vi "CC Observation Queue GUI.vi"() -> ()   [LabVIEW 2024]
uses:
  Subsystems/SS cluster Script Status Queue.ctl
  typedefs/CC cluster Observation.ctl
  CC enum Observation Status.ctl
  Telescope/CC cluster Telescope Offsets.ctl
  typedefs/CC cluster Observation Dither Options.ctl
  typedefs/CC enum Dither Selection.ctl
  typedefs/CC cluster RA and DEC.ctl
  Subsystems/SS typedef cluster Instrument Command Queue Data.ctl
  CC cluster Script State.ctl
  CC cluster Observation Settings.ctl
  CC cluster Air Mass Data.ctl
  Logging/CC enum Current Values Action.ctl
  typedefs/CC cluster Script.ctl
  typedefs/CC Script Step.ctl
  typedefs/CC enum Script Action.ctl
  Scripts/CC Rd Wr Script Action.ctl
  typedefs/CC enum Alarm Action.ctl
  hk-channel-class/hk-channel-class/HK Table/HK Table.lvclass
panel:
  in  "Open Plots":bool
  in  "Air Mass Tool":bool
  out "Row":i32 caption="Next"
  in  "queue idle":string="TELESCOPE IDLE"
  in  "clean table":bool
  in  "Auto Step":bool
  in  "Stop":bool
  out "Queue Running":i16(slide) scale=-1.0..4.0
  in  "Pause Q":bool
  in  "Run Queue":bool
  in  "Close":bool
  out "Queue":i32(listbox)
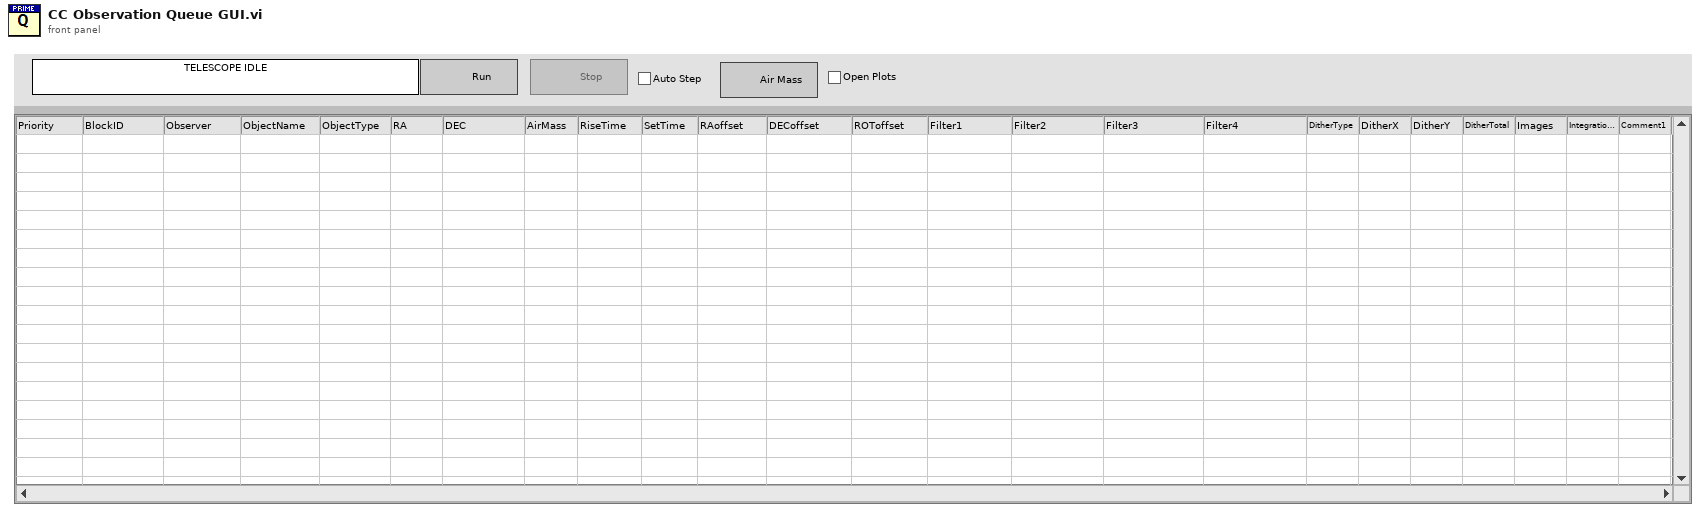
[diagram p1: front panel]
types:
  T1 = typedef "CC cluster Observation.ctl" = cluster{"Priority":i32, "ID":string, "Observer":string, "Obj Name":string, "Obj Type":string, "RA and DEC String":cluster{"RA":string, "DEC":string}, "Filters":string[], "Integration Time":dbl, "Observation Status":T2, "Offsets":T3, "Images":i32, "Dither Options":T4, "Comment 1":string, "Comment 2":string}
  T2 = typedef "CC enum Observation Status.ctl" = enum16{"Ready", "Running", "Done", "Error"}
  T3 = typedef "CC cluster Telescope Offsets.ctl" = cluster{"RA":dbl, "DEC":dbl, "ROT":dbl}
  T4 = typedef "CC cluster Observation Dither Options.ctl" = cluster{"Dither":T5, "Dither Radius":dbl, "Dither Points":i32, "Dither Phase":dbl, "B Offset":T6}
  T5 = typedef "CC enum Dither Selection.ctl" = enum16{"None", "Circle", "Random", "ABBA"}
  T6 = typedef "CC cluster RA and DEC.ctl" = cluster{"RA":dbl, "DEC":dbl}
  T7 = typedef "CC cluster Script State.ctl" = cluster{"Image Count":i32, "Step":i32, "Dither Idx":i32, "Dither Total":i32, "Running":bool, "State":u16}
  T8 = typedef "CC cluster Observation Settings.ctl" = cluster{"Air Mass Program Path":path}
  T9 = typedef "CC cluster Air Mass Data.ctl" = cluster{"BlockID":string, "Air Mass":string, "Rise Time":string, "Set Time":string}
  T10 = cluster{"state":refnum<user-event>, "Obs Queue":refnum<queue>, "Observation List":T1[], "Data":variant, "Obs State":enum16{"Idle", "Running", "Paused"}, "Row":i32, "Script Q":refnum<queue>, "Expected Images":i32, "Script Status":T7, "Prev Status":T7, "script name":string, "Observation Settings":T8, "BlockIDs":string[], "Airmass Idx":i32, "Air Mass":T9[]}
  T11 = typedef "CC enum Current Values Action.ctl" = enum16{"Init", "Write Item", "Write Array", "Read Item", "Read Array", "Read All", "Add Channels", "New File", "Add Message", "Get Current Values", "Close"}
  T12 = enum8{"Enabled", "Disabled", "Disabled and Grayed Out"}
  T13 = typedef "CC Rd Wr Script Action.ctl" = enum16{"Read", "Write", "List", "Delete"}
  T14 = typedef "CC cluster Script.ctl" = cluster{"Name":string, "Script":T15[]}
  T15 = typedef "CC Script Step.ctl" = cluster{"Action":T16, "Data":variant}
  T16 = typedef "CC enum Script Action.ctl" = enum16{"Noop", "Define Object", "Define Exposure", "Define Dithering", "Acquire Images", "Set Filter Wheel", "Telescope Home", "Telescope Move", "Telescope RA DEC", "Focus Move Relative", "Focus Move Absolute", "Focus Set Home", "Macro", "Pause", "Ask User", "Define Random Dither", "CmdLine", "Outlet"}
  T17 = typedef "SS typedef cluster Instrument Command Queue Data.ctl" = cluster{"Cmd":string, "Parameters":variant}
  T18 = typedef "CC enum Alarm Action.ctl" = enum16{"Init", "Add Alarm", "Get Alarms", "Clear Alarm", "Clear All Alarms"}
  T19 = typedef "SS cluster Script Status Queue.ctl" = cluster{"Msg":string, "Data":variant}
  T20 = typedef "CC cluster Script Panel Defaults.ctl" = cluster{"Script Name":string, "Script Path":path}
  T21 = typedef "LVPoint32TypeDef.ctl" = cluster{"Horizontal":i32, "Vertical":i32}
  T22 = typedef "LVRowAndColumnTypeDef.ctl" = cluster{"Row":i32, "Column":i32}
  T23 = typedef "CC cluster Alarm Data.ctl" = cluster{"Measured Value":dbl, "Alarm Low":dbl, "Alarm High":dbl, "Message":string, "Source":string}
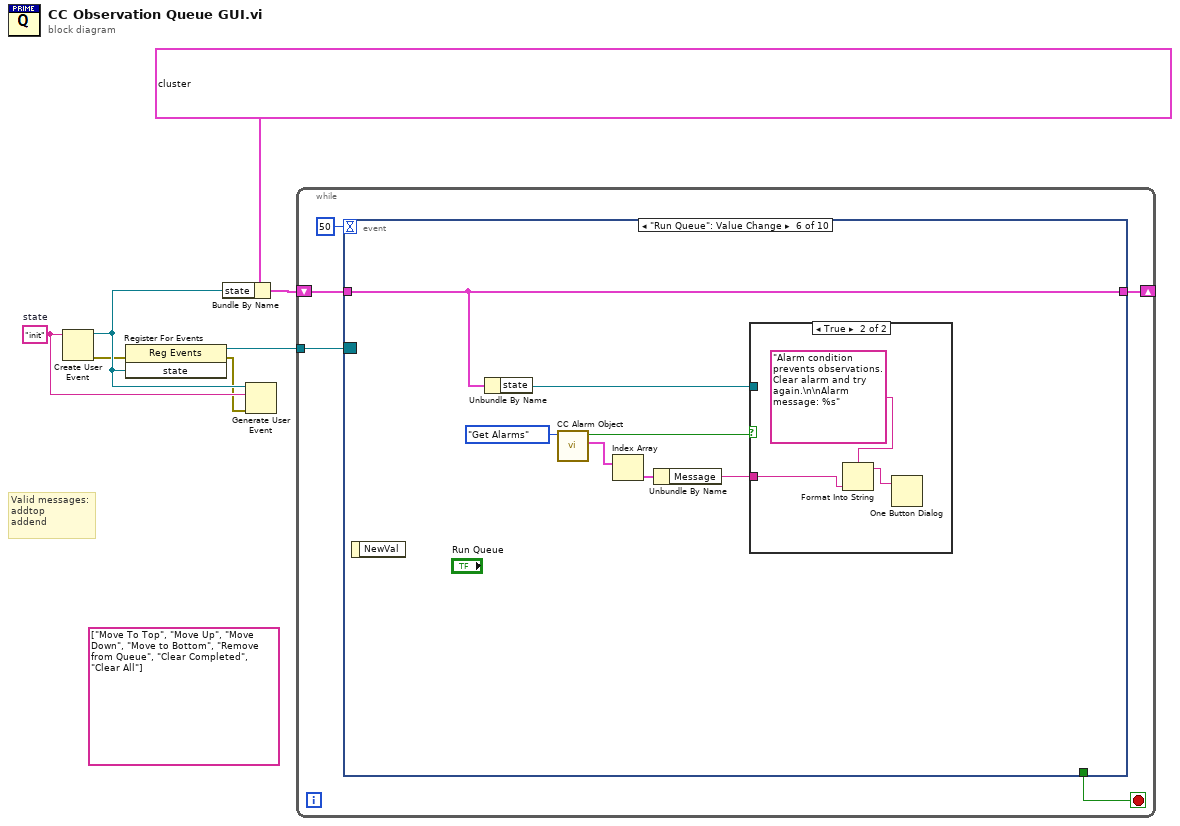
[diagram p0: block diagram]
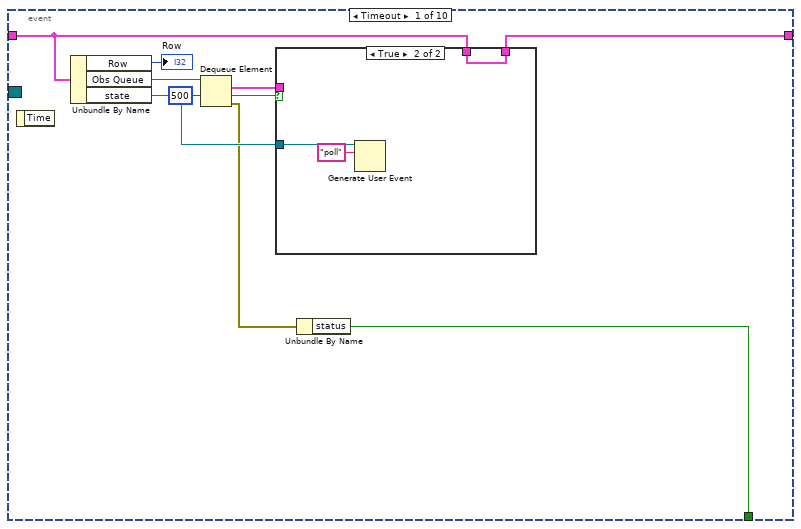
[diagram p2: hidden frame]
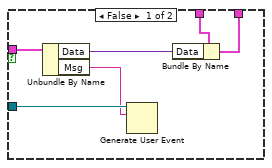
[diagram p3: hidden frame]
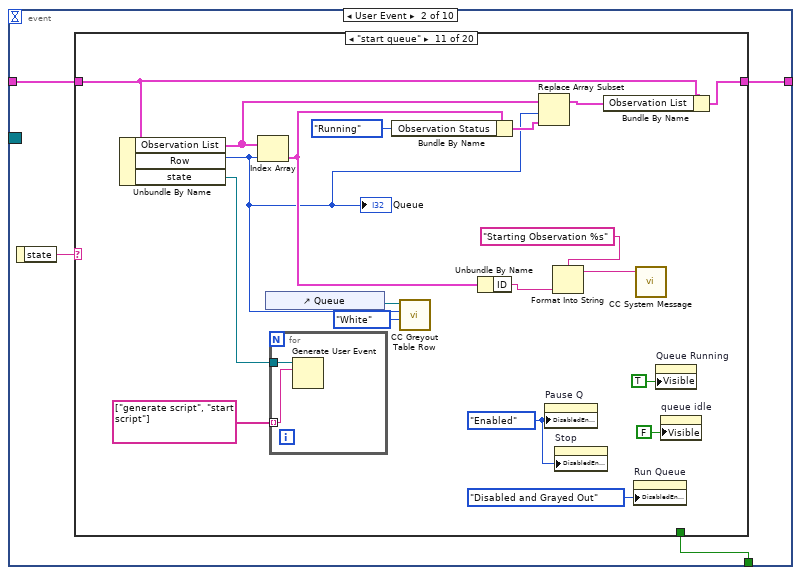
[diagram p4: hidden frame]
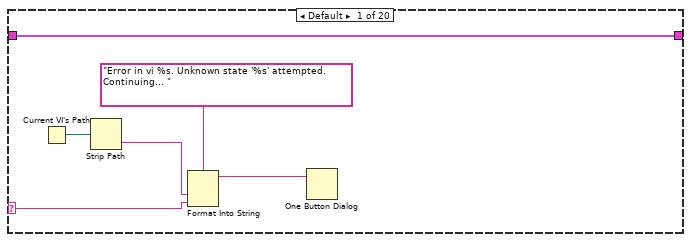
[diagram p5: hidden frame]
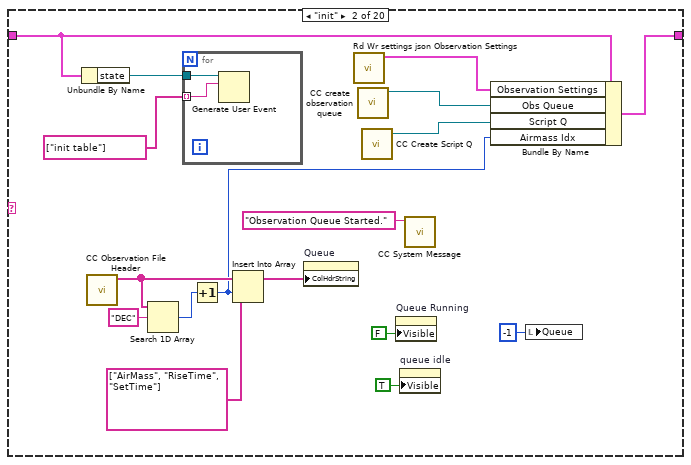
[diagram p6: hidden frame]
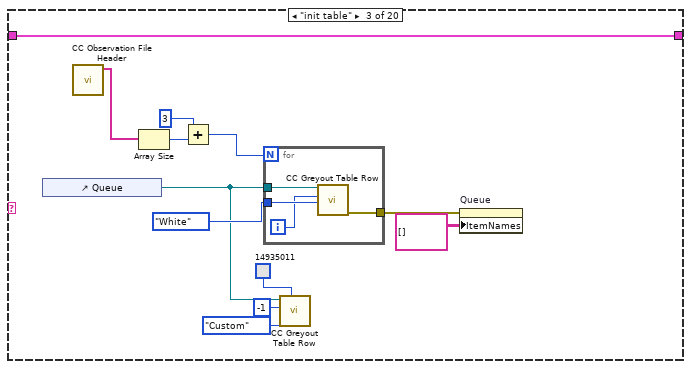
[diagram p7: hidden frame]
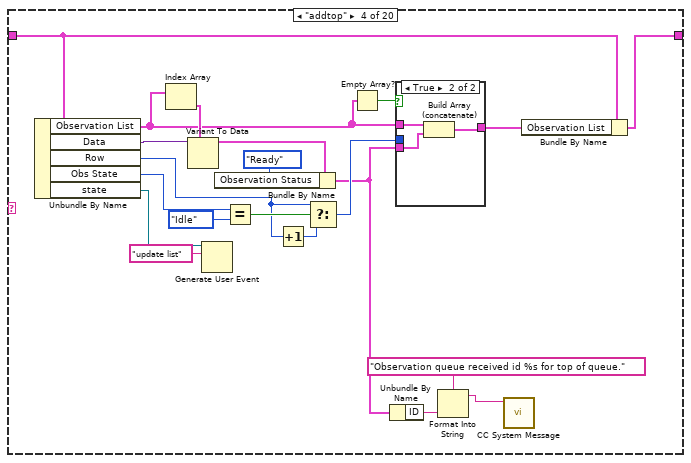
[diagram p8: hidden frame]
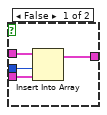
[diagram p9: hidden frame]
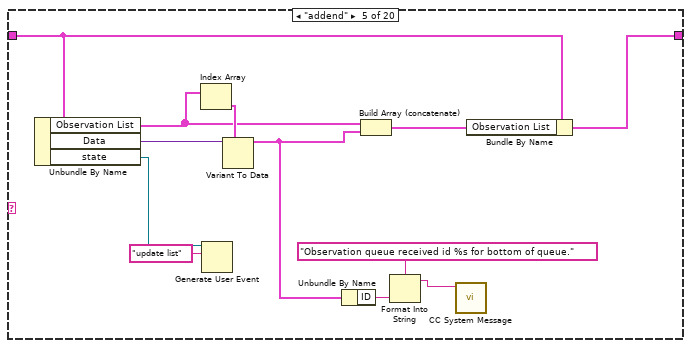
[diagram p10: hidden frame]
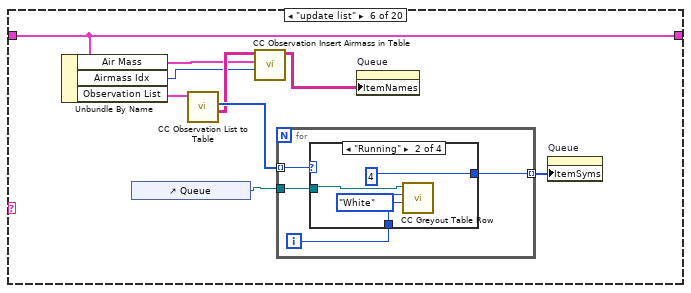
[diagram p11: hidden frame]
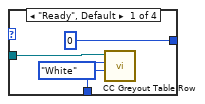
[diagram p12: hidden frame]
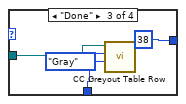
[diagram p13: hidden frame]
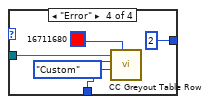
[diagram p14: hidden frame]
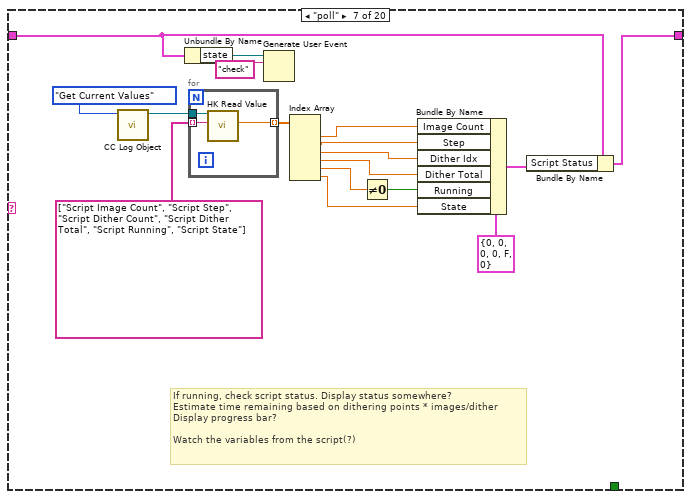
[diagram p15: hidden frame]
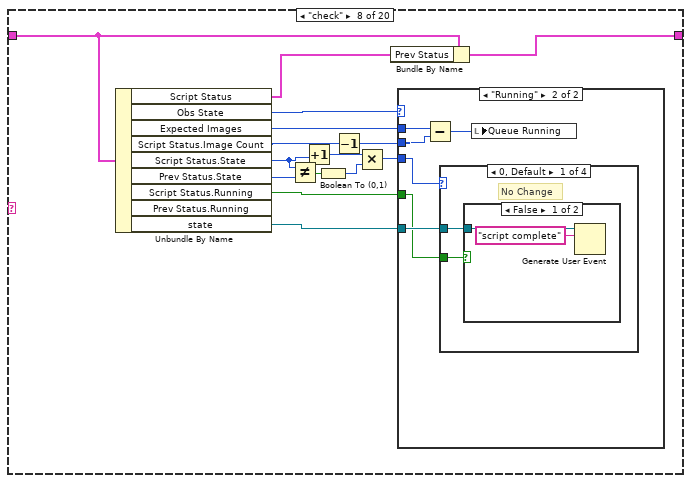
[diagram p16: hidden frame]
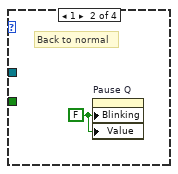
[diagram p19: hidden frame]
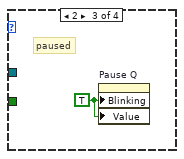
[diagram p20: hidden frame]
diagram:
  (unwired) string[] ["Move To Top", "Move Up", "Move Down", "Move to Bottom", "Remove from Queue", "Clear Completed", "Clear All"]
  w3 = "init"  # state
  # "Valid messages:\naddtop\naddend"
  n1 = Create User Event(user event datatype=w3) -> (user event=w5:refnum<user-event>, error out=w1:errorcluster)  [unwired: 1 in]
  n2 = register-events(error in=w1, w5) -> (reference out=w4:refnum<event-registration>, error out=w2:errorcluster)  [unwired: 1 in]
  n3 = Bundle By Name(cluster=T10 {"state"=refnum, "Obs Queue"=refnum, "Observation List"=[], "Data"=variant, "Obs State"=enum."Idle", "Row"=0, "Script Q"=refnum, "Expected Images"=0, "Script Status"={"Image Count"=0, "Step"=0, "Dither Idx"=0, "Dither Total"=0, "Running"=FALSE, "State"=0}, "Prev Status"={"Image Count"=0, "Step"=0, "Dither Idx"=0, "Dither Total"=0, "Running"=FALSE, "State"=0}, "script name"="", "Observation Settings"={"Air Mass Program Path"=path ""}, "BlockIDs"=["P0102", "P00002", "P00003", "P00004", "P00005", "P00006"], "Airmass Idx"=0, "Air Mass"=[{"BlockID"="", "Air Mass"="", "Rise Time"="06:16", "Set Time"="13:33"}, {"BlockID"="", "Air Mass"="", "Rise Time"="06:16", "Set Time"="13:33"}, {"BlockID"="", "Air Mass"="", "Rise Time"="06:16", "Set Time"="13:33"}, {"BlockID"="", "Air Mass"="", "Rise Time"="06:16", "Set Time"="13:33"}, {"BlockID"="", "Air Mass"="", "Rise Time"="06:16", "Set Time"="13:33"}, {"BlockID"="", "Air Mass"="", "Rise Time"="06:16", "Set Time"="13:33"}]}, "state"=w5) -> (w6:T10)
  n4 = Generate User Event(user event=w5, event data cluster=w3, error in=w2) -> ()  [unwired: 1 in, 2 out]
  n5 = while {
    tunnel: w4 -> [w12]
    shift-right: [w10] -> _
    shift-left: w6 -> [w11]
    stop <- w9 stop-if-true
    n6 = event shown="[5] \"Run Queue\": Value Change" {
      selector: w12 -> [_ _ _ _ _ _ _ _ _ _]
      dyn-events: _ -> [_ _ _ _ _ _ _ _ _ _]
      timeout: 50 -> [_ _ _ _ _ _ _ _ _ _]
      tunnel: w11 -> [w17 w34 w400 w432 w501 w578 w589 w594 w598 w600]
      tunnel: [w18 w33 w401 w432 w502 w578 w589 w594 w598 w600] -> w10
      tunnel: [w14 w32 _ _ _ _ _ _ _ "Close"] -> w9
      event Timeout {
        n7 = event-data() -> ()  [unwired: 1 in, 1 out]
        n8 = Unbundle By Name(w17) -> ("Row"=→"Row":i32, "Obs Queue"=w22:refnum<queue>, "state"=w19:refnum<user-event>)
        n9 = Dequeue Element(queue=w22, timeout in ms (-1)=500) -> (element=w20:T19, timed out?=w21:bool, error out=w15:errorcluster)  [unwired: 1 in, 1 out]
        n10 = case shown="True" w21 {
          tunnel: w20 -> [w28 _]
          tunnel: w19 -> [w27 w30]
          tunnel: w17 -> [w25 w31]
          tunnel: [w23 w31] -> w18
          frame False {
            n11 = Unbundle By Name(w28) -> ("Data"=w24:variant, "Msg"=w26:string)
            n12 = Generate User Event(user event=w27, event data cluster=w26) -> ()  [unwired: 2 in, 2 out]
            n13 = Bundle By Name(cluster=w25, "Data"=w24) -> (w23:T10)
          }
          frame True {
            n14 = Generate User Event(user event=w30, event data cluster="poll" ("event data")) -> ()  [unwired: 2 in, 2 out]
          }
        }
        n15 = Unbundle By Name(w15) -> ("status"=w14:bool)
      }
      event User Event {
        n16 = event-data() -> ("state"=w35:string)  [unwired: 1 in]
        n17 = case shown="\"start queue\"" w35 {
          selector: w35 -> [w40 _ _ _ _ _ _ _ _ _ _ _ _ _ _ _ _ _ _ _]
          tunnel: w34 -> [w36 w54 w72 w93 w111 w125 w150 w168 w202 w228 w232 w255 w293 w316 w337 w357 w366 w382 w392 w397]
          tunnel: [w36 w57 w72 w94 w112 w125 w151 w169 w203 w229 w233 w256 w304 w317 w338 w357 w367 w383 w392 w397] -> w33
          tunnel: [_ _ _ _ _ _ _ _ _ _ _ _ _ _ _ _ _ _ _ TRUE] -> w32
          frame Default {
            n18 = Current VI's Path() -> (path=w39:path)
            n19 = Strip Path(path=w39) -> (name=w38:string)  [unwired: 1 out]
            n20 = Format Into String(format string="Error in vi %s. Unknown state '%s' attempted. Continuing... ", w38, w40) -> (resulting string=w37:string)  [unwired: 2 in, 1 out]
            n21 = One Button Dialog(message=w37) -> ()  [unwired: 1 in, 1 out]
          }
          frame "init" {
            n22 = Unbundle By Name(w54) -> ("state"=w53:refnum<user-event>)
            n23 = call "CC Observation File Header.vi"() -> ("Header"=w47:string[])  [unwired: 10 in, 1 out]
            n24 = Search 1D Array(1D array=w47, element="DEC") -> (index of element=w44:i32)  [unwired: 1 in]
            n25 = for {
              tunnel: w53 -> [w60]
              tunnel: string[] ["init table"] -> [w59] mode=indexing
              n26 = Generate User Event(user event=w60, event data cluster=w59) -> ()  [unwired: 2 in, 2 out]
            }
            n27 = Increment(x=w44) -> (x+1=w42:i32)
            n28 = Insert Into Array(array=w47, index=w42, new element=string[] ["AirMass", "RiseTime", "SetTime"]) -> (w45:string[])
            n29 = property on="Queue" class="MCListbox (strict)"("ColHdrString"=w45) -> ()  [unwired: 2 in, 2 out]
            n30 = call "Rd Wr settings json Observation Settings.vi"() -> ("Observation Settings"=w48:T8)  [unwired: 10 in, 1 out]
            n31 = call "CC create observation queue.vi"() -> ("Observation Queue"=w58:refnum<queue>)  [unwired: 10 in, 1 out]
            n32 = call "CC Create Script Q.vi"() -> ("Script Q"=w56:refnum<queue>)  [unwired: 10 in, 1 out]
            n33 = property on="Queue Running" class="Slide (strict)"("Visible"=FALSE) -> ()  [unwired: 2 in, 2 out]
            n34 = property on="queue idle" class="Str"("Visible"=TRUE) -> ()  [unwired: 2 in, 2 out]
            n35 = call "CC System Message.vi"("Message"="Observation Queue Started.") -> ()  [unwired: 10 in, 1 out]
            n36 = Bundle By Name(cluster=w54, "Observation Settings"=w48, "Obs Queue"=w58, "Script Q"=w56, "Airmass Idx"=w42) -> (w57:T10)
            n37 = local write "Queue"(-1 ("Queue")) -> ()
          }
          frame "init table" {
            n38 = control-ref of="Queue"() -> (w68:refnum<vi>)
            n39 = call "CC Observation File Header.vi"() -> ("Header"=w64:string[])  [unwired: 10 in, 1 out]
            n40 = Array Size(array=w64) -> (size(s)=w63:i32)
            n41 = Add(x=3, y=w63) -> (x+y=w62:i32)
            n42 = for {
              N: w62 -> [_]
              tunnel: w68 -> [w76]
              tunnel: [w75] -> w71
              tunnel: enum16{"White", "Gray", "Custom"}."White" ("Color") -> [w74]
              i -> [w73]
              n43 = call "CC Greyout Table Row.vi"("Color"=w74, "Row"=w73, "Queue ref"=w76) -> ("error out"=w75:errorcluster)  [unwired: 8 in]
            }
            n44 = call "CC Greyout Table Row.vi"("Color Box"=u32 14935011, "Color"=enum16{"White", "Gray", "Custom"}."Custom", "Row"=-1, "Queue ref"=w68) -> ()  [unwired: 7 in, 1 out]
            n45 = property on="Queue" class="MCListbox (strict)"(error in=w71, "ItemNames"=string[][] [] ("Item Names")) -> ()  [unwired: 1 in, 2 out]
          }
          frame "addtop" {
            n46 = Unbundle By Name(w93) -> ("Observation List"=w82:T1[], "Data"=w97:variant, "Row"=w77:i32, "Obs State"=w92:enum16{"Idle", "Running", "Paused"}, "state"=w87:refnum<user-event>)
            n47 = Index Array(array=w82) -> (element=w96:T1)  [unwired: 1 in]
            n48 = Variant To Data(type=w96, Variant=w97) -> (data=w81:T1)  [unwired: 1 in, 1 out]
            n49 = Generate User Event(user event=w87, event data cluster="update list" ("event data")) -> ()  [unwired: 2 in, 2 out]
            n50 = Bundle By Name(cluster=w81, "Observation Status"=CC_enum_Observation_Status."Ready") -> (w79:T1)
            n51 = Equal?(x=w92, y=enum16{"Idle", "Running", "Paused"}."Idle") -> (x = y?=w90:bool)
            n52 = Increment(x=w77) -> (x+1=w88:i32)
            n53 = Select(t=w77, s=w90, f=w88) -> (s? t:f=w89:i32)
            n54 = Empty Array?(array=w82) -> (empty?=w78:bool)
            n55 = Unbundle By Name(w79) -> ("ID"=w84:string)
            n56 = case shown="True" w78 {
              tunnel: [w101 w102] -> w95
              tunnel: w89 -> [w100 _]
              tunnel: w82 -> [w99 w104]
              tunnel: w79 -> [w98 w103]
              frame False {
                n57 = Insert Into Array(array=w99, index=w100, new element=w98) -> (w101:T1[])
              }
              frame True {
                n58 = Build Array (concatenate)(w104, w103) -> (w102:T1[])
              }
            }
            n59 = Format Into String(format string="Observation queue received id %s for top of queue.", w84) -> (resulting string=w83:string)  [unwired: 2 in, 1 out]
            n60 = call "CC System Message.vi"("Message"=w83) -> ()  [unwired: 10 in, 1 out]
            n61 = Bundle By Name(cluster=w93, "Observation List"=w95) -> (w94:T10)
          }
          frame "addend" {
            n62 = Unbundle By Name(w111) -> ("Observation List"=w114:T1[], "Data"=w116:variant, "state"=w110:refnum<user-event>)
            n63 = Index Array(array=w114) -> (element=w115:T1)  [unwired: 1 in]
            n64 = Generate User Event(user event=w110, event data cluster="update list" ("event data")) -> ()  [unwired: 2 in, 2 out]
            n65 = Variant To Data(type=w115, Variant=w116) -> (data=w105:T1)  [unwired: 1 in, 1 out]
            n66 = Unbundle By Name(w105) -> ("ID"=w107:string)
            n67 = Build Array (concatenate)(w114, w105) -> (w113:T1[])
            n68 = Format Into String(format string="Observation queue received id %s for bottom of queue.", w107) -> (resulting string=w106:string)  [unwired: 2 in, 1 out]
            n69 = call "CC System Message.vi"("Message"=w106) -> ()  [unwired: 10 in, 1 out]
            n70 = Bundle By Name(cluster=w111, "Observation List"=w113) -> (w112:T10)
          }
          frame "update list" {
            n71 = Unbundle By Name(w125) -> ("Air Mass"=w119:T9[], "Airmass Idx"=w118:i32, "Observation List"=w124:T1[])
            n72 = control-ref of="Queue"() -> (w121:refnum<vi>)
            n73 = call "CC Observation List to Table.vi"("Observation List"=w124) -> ("Screen Ready Table"=w120:string[][], "Status"=w123:T2[])  [unwired: 7 in, 2 out]
            n74 = call "CC Observation Insert Airmass in Table.vi"("Airmass Idx"=w118, "Air Mass"=w119, "Table"=w120) -> ("Table out"=w117:string[][])  [unwired: 8 in]
            n75 = for {
              tunnel: w123 -> [w129] mode=indexing
              tunnel: [w128] -> w122 mode=indexing
              tunnel: w121 -> [w126]
              i -> [w127]
              n76 = case shown="\"Running\"" w129 {
                tunnel: [0 4 ("new element/subarray") 38 ("new element/subarray") 2 ("new element/subarray")] -> w128
                tunnel: w127 -> [w132 w137 w140 w143]
                tunnel: w126 -> [w130 w136 w139 w145]
                frame "Ready", Default {
                  n77 = call "CC Greyout Table Row.vi"("Color"=enum16{"White", "Gray", "Custom"}."White", "Row"=w132, "Queue ref"=w130) -> ()  [unwired: 8 in, 1 out]
                }
                frame "Running" {
                  n78 = call "CC Greyout Table Row.vi"("Color"=enum16{"White", "Gray", "Custom"}."White", "Row"=w137, "Queue ref"=w136) -> ()  [unwired: 8 in, 1 out]
                }
                frame "Done" {
                  n79 = call "CC Greyout Table Row.vi"("Color"=enum16{"White", "Gray", "Custom"}."Gray", "Row"=w140, "Queue ref"=w139) -> ()  [unwired: 8 in, 1 out]
                }
                frame "Error" {
                  n80 = call "CC Greyout Table Row.vi"("Color Box"=u32 16711680, "Color"=enum16{"White", "Gray", "Custom"}."Custom", "Row"=w143, "Queue ref"=w145) -> ()  [unwired: 7 in, 1 out]
                }
              }
            }
            n81 = property on="Queue" class="MCListbox (strict)"("ItemNames"=w117) -> ()  [unwired: 2 in, 2 out]
            n82 = property on="Queue" class="MCListbox (strict)"("ItemSyms"=w122) -> ()  [unwired: 2 in, 2 out]
          }
          frame "poll" {
            # "If running, check script status. Display status somewhere?\nEstimate time remaining based on dithering points * images/dither\nDisplay progress bar?\n\nWatch the variables from the script(?)"
            n83 = call "CC Log Object.vi"("Action"=CC_enum_Current_Values_Action."Get Current Values") -> ("HK Channel out"=w162:refnum<class "HK Table.lvclass">)  [unwired: 8 in, 2 out]
            n84 = Unbundle By Name(w150) -> ("state"=w148:refnum<user-event>)
            n85 = for {
              tunnel: w162 -> [w166]
              tunnel: string[] ["Script Image Count", "Script Step", "Script Dither Count", "Script Dither Total", "Script Running", "Script State"] -> [w165] mode=indexing
              tunnel: [w164] -> w161 mode=indexing
              n86 = call-dynamic "HK Read Value.vi"("Channel Name"=w165, "HK Channel in"=w166) -> ("Value"=w164:dbl)  [unwired: 4 in, 5 out]
            }
            n87 = Generate User Event(user event=w148, event data cluster="check" ("event data")) -> ()  [unwired: 2 in, 2 out]
            n88 = Index Array(array=w161) -> (element #1=w149:dbl, element #2=w158:dbl, element #3=w157:dbl, element #4=w156:dbl, element #5=w155:dbl, element #6=w153:dbl)  [unwired: 6 in]
            n89 = Not Equal To 0?(x=w155) -> (x != 0?=w154:bool)
            n90 = Bundle By Name(cluster=T7 {"Image Count"=0, "Step"=0, "Dither Idx"=0, "Dither Total"=0, "Running"=FALSE, "State"=0}, "Image Count"=w149, "Step"=w158, "Dither Idx"=w157, "Dither Total"=w156, "Running"=w154, "State"=w153) -> (w152:T7)
            n91 = Bundle By Name(cluster=w150, "Script Status"=w152) -> (w151:T10)
          }
          frame "check" {
            n92 = Unbundle By Name(w168) -> ("Script Status"=w170:T7, "Obs State"=w181:enum16{"Idle", "Running", "Paused"}, "Expected Images"=w180:i32, "Script Status.Image Count"=w179:i32, "Script Status.State"=w177:u16, "Prev Status.State"=w178:u16, "Script Status.Running"=w171:bool, "state"=w172:refnum<user-event>)  [unwired: 1 out]
            n93 = Not Equal?(x=w177, y=w178) -> (x != y?=w175:bool)
            n94 = Increment(x=w177) -> (x+1=w176:u16)
            n95 = Boolean To (0,1)(Boolean=w175) -> (0, 1=w173:i16)
            n96 = Decrement(x=w179) -> (x-1=w167:i32)
            n97 = Multiply(x=w176, y=w173) -> (x*y=w174:u16)
            n98 = Bundle By Name(cluster=w168, "Prev Status"=w170) -> (w169:T10)
            n99 = case shown="\"Running\"" w181 {
              tunnel: w180 -> [_ w187]
              tunnel: w167 -> [_ w185]
              tunnel: w174 -> [_ w184]
              tunnel: w172 -> [_ w183]
              tunnel: w171 -> [_ w182]
              frame "Idle", Default {
              }
              frame "Running" {
                n100 = Subtract(x=w187, y=w185) -> (x-y=w186:i32)
                n101 = case shown="0, Default" w184 {
                  tunnel: w183 -> [w189 _ _ w195]
                  tunnel: w182 -> [w188 _ _ _]
                  frame 0, Default {
                    # "No Change"
                    n102 = case shown="False" w188 {
                      tunnel: w189 -> [w190 _]
                      frame False {
                        n103 = Generate User Event(user event=w190, event data cluster="script complete" ("event data")) -> ()  [unwired: 2 in, 2 out]
                      }
                      frame True {
                      }
                    }
                  }
                  frame 1 {
                    w192 = FALSE ("Blinking")
                    # "Back to normal"
                    n104 = property on="Pause Q" class="Bool (strict)"("Blinking"=w192, "Value"=w192) -> ()  [unwired: 2 in, 2 out]
                  }
                  frame 2 {
                    w193 = TRUE ("Blinking")
                    # "paused"
                    n105 = property on="Pause Q" class="Bool (strict)"("Blinking"=w193, "Value"=w193) -> ()  [unwired: 2 in, 2 out]
                  }
                  frame 3 {
                    # "Error"
                    n106 = Generate User Event(user event=w195, event data cluster="script error" ("event data")) -> ()  [unwired: 2 in, 2 out]
                  }
                }
                n107 = local write "Queue Running"(w186) -> ()
              }
            }
          }
          frame "add to top" {
            n108 = Unbundle By Name(w202) -> ("Data"=w209:variant, "Obs State"=w208:enum16{"Idle", "Running", "Paused"}, "Row"=w207:i32, "Observation List"=w206:T1[], "state"=w201:refnum<user-event>)
            n109 = Variant To Data(type=T1 {"Priority"=0, "ID"="", "Observer"="", "Obj Name"="", "Obj Type"="", "RA and DEC String"={"RA"="", "DEC"=""}, "Filters"=[], "Integration Time"=0.0, "Observation Status"=enum."Error", "Offsets"={"RA"=0.0, "DEC"=0.0, "ROT"=0.0}, "Images"=0, "Dither Options"={"Dither"=enum."Random", "Dither Radius"=0.0, "Dither Points"=0, "Dither Phase"=0.0, "B Offset"={"RA"=0.0, "DEC"=0.0}}, "Comment 1"="", "Comment 2"=""} ("Observation"), Variant=w209) -> (data=w205:T1)  [unwired: 1 in, 1 out]
            n110 = Generate User Event(user event=w201, event data cluster="update list" ("event data")) -> ()  [unwired: 2 in, 2 out]
            n111 = case shown="\"Idle\", Default" w208 {
              tunnel: w207 -> [_ w219]
              tunnel: w206 -> [w214 w218]
              tunnel: w205 -> [w211 w215]
              tunnel: [w212 w216] -> w204
              tunnel: [w211 w215] -> w198
              frame "Idle", Default {
                n112 = Insert Into Array(array=w214, index=0, new element=w211) -> (w212:T1[])
              }
              frame "Running", "Paused" {
                n113 = Increment(x=w219) -> (x+1=w217:i32)
                n114 = Insert Into Array(array=w218, index=w217, new element=w215) -> (w216:T1[])
              }
            }
            n115 = Unbundle By Name(w198) -> ("ID"=w197:string)
            n116 = Format Into String(format string="Observation ID %s added to top of Queue" ("Message"), w197) -> (resulting string=w196:string)  [unwired: 2 in, 1 out]
            n117 = Bundle By Name(cluster=w202, "Observation List"=w204) -> (w203:T10)
            n118 = call "CC System Message.vi"("Message"=w196) -> ()  [unwired: 10 in, 1 out]
          }
          frame "add to bottom" {
            n119 = Unbundle By Name(w228) -> ("Data"=w230:variant, "Observation List"=w225:T1[], "state"=w227:refnum<user-event>)
            n120 = Variant To Data(type=T1 {"Priority"=0, "ID"="", "Observer"="", "Obj Name"="", "Obj Type"="", "RA and DEC String"={"RA"="", "DEC"=""}, "Filters"=[], "Integration Time"=0.0, "Observation Status"=enum."Error", "Offsets"={"RA"=0.0, "DEC"=0.0, "ROT"=0.0}, "Images"=0, "Dither Options"={"Dither"=enum."Random", "Dither Radius"=0.0, "Dither Points"=0, "Dither Phase"=0.0, "B Offset"={"RA"=0.0, "DEC"=0.0}}, "Comment 1"="", "Comment 2"=""} ("Observation"), Variant=w230) -> (data=w220:T1)  [unwired: 1 in, 1 out]
            n121 = Generate User Event(user event=w227, event data cluster="update list" ("event data")) -> ()  [unwired: 2 in, 2 out]
            n122 = Build Array (concatenate)(w225, w220) -> (w224:T1[])
            n123 = Unbundle By Name(w220) -> ("ID"=w222:string)
            n124 = Format Into String(format string="Observation ID %s added to end of Queue" ("Message"), w222) -> (resulting string=w221:string)  [unwired: 2 in, 1 out]
            n125 = Bundle By Name(cluster=w228, "Observation List"=w224) -> (w229:T10)
            n126 = call "CC System Message.vi"("Message"=w221) -> ()  [unwired: 10 in, 1 out]
          }
          frame "start queue" {
            w247 = T12."Enabled" ("Disabled")
            n127 = Unbundle By Name(w232) -> ("Observation List"=w237:T1[], "Row"=w235:i32, "state"=w249:refnum<user-event>)
            "Queue" <- w235
            n128 = Index Array(array=w237, index=w235) -> (element=w239:T1)
            n129 = control-ref of="Queue"() -> (w243:refnum<vi>)
            n130 = for {
              tunnel: w249 -> [w252]
              tunnel: string[] ["generate script", "start script"] -> [w251] mode=indexing
              n131 = Generate User Event(user event=w252, event data cluster=w251) -> ()  [unwired: 2 in, 2 out]
            }
            n132 = Bundle By Name(cluster=w239, "Observation Status"=CC_enum_Observation_Status."Running") -> (w236:T1)
            n133 = call "CC Greyout Table Row.vi"("Color"=enum16{"White", "Gray", "Custom"}."White", "Row"=w235, "Queue ref"=w243) -> ()  [unwired: 8 in, 1 out]
            n134 = Unbundle By Name(w239) -> ("ID"=w245:string)
            n135 = Replace Array Subset(array=w237, new element=w236, index=w235) -> (w234:T1[])
            n136 = property on="Pause Q" class="Bool (strict)"("DisabledEnum"=w247) -> ()  [unwired: 2 in, 2 out]
            n137 = Format Into String(format string="Starting Observation %s" ("Message"), w245) -> (resulting string=w244:string)  [unwired: 2 in, 1 out]
            n138 = property on="Stop" class="Bool"("DisabledEnum"=w247) -> ()  [unwired: 2 in, 2 out]
            n139 = Bundle By Name(cluster=w232, "Observation List"=w234) -> (w233:T10)
            n140 = property on="Run Queue" class="Bool"("DisabledEnum"=T12."Disabled and Grayed Out" ("Disabled")) -> ()  [unwired: 2 in, 2 out]
            n141 = call "CC System Message.vi"("Message"=w244) -> ()  [unwired: 10 in, 1 out]
            n142 = property on="Queue Running" class="Slide (strict)"("Visible"=TRUE) -> ()  [unwired: 2 in, 2 out]
            n143 = property on="queue idle" class="Str"("Visible"=FALSE) -> ()  [unwired: 2 in, 2 out]
          }
          frame "quick image" {
            n144 = Unbundle By Name(w255) -> ("state"=w253:refnum<user-event>, "Obs State"=w254:enum16{"Idle", "Running", "Paused"}, "Script Q"=w257:refnum<queue>, "Data"=w258:variant)
            n145 = case shown="\"Idle\"" w254 {
              tunnel: w258 -> [w281 _]
              tunnel: w257 -> [w277 _]
              tunnel: [w262 w283] -> w256
              tunnel: w255 -> [w261 w283]
              tunnel: w253 -> [w260 _]
              frame "Idle" {
                n146 = Variant To Data(type=T1 {"Priority"=0, "ID"="", "Observer"="", "Obj Name"="", "Obj Type"="", "RA and DEC String"={"RA"="HH:MM:SS.nnn", "DEC"="DEG:arcmin:arcsec.nn"}, "Filters"=[], "Integration Time"=0.0, "Observation Status"=enum."Error", "Offsets"={"RA"=0.0, "DEC"=0.0, "ROT"=0.0}, "Images"=0, "Dither Options"={"Dither"=enum."None", "Dither Radius"=0.0, "Dither Points"=0, "Dither Phase"=0.0, "B Offset"={"RA"=0.0, "DEC"=0.0}}, "Comment 1"="", "Comment 2"=""} ("element"), Variant=w281) -> (data=w275:T1)  [unwired: 1 in, 1 out]
                n147 = Format Date/Time String(time format string (%c)="%Y%m%d_%H%M%S") -> (date/time string=w265:string)  [unwired: 2 in]
                n148 = call "CC Observation to Script.vi"("Observation"=w275) -> ("Script Steps"=w264:T15[])  [unwired: 9 in, 1 out]
                n149 = call "Rd Wr Script Defaults.vi"() -> ("Script Settings"=w272:T20)  [unwired: 10 in, 1 out]
                n150 = Format Into String(format string="QuickObs_%s", w265) -> (resulting string=w263:string)  [unwired: 2 in, 1 out]
                n151 = Bundle(cluster=T17 {"Cmd"="", "Parameters"=variant} ("element"), "Cmd"="set observation", "Parameters"=w275) -> (w276:T17)
                n152 = Unbundle By Name(w272) -> ("Script Path"=w271:path)
                n153 = Bundle By Name(cluster=T14 {"Name"="", "Script"=[]} ("Script"), "Name"=w263, "Script"=w264) -> (w273:T14)
                n154 = Generate User Event(user event=w260, event data cluster="start script" ("event data")) -> ()  [unwired: 2 in, 2 out]
                n155 = Enqueue Element(queue=w277, element=w276) -> ()  [unwired: 2 in, 3 out]
                n156 = Bundle By Name(cluster=w261, "script name"=w263) -> (w262:T10)
                n157 = Format Into String(format string="Created script %s.", w263) -> (resulting string=w267:string)  [unwired: 2 in, 1 out]
                n158 = call "CC Rd Wr Script.vi"("Script Path"=w271, "Action"=CC_Rd_Wr_Script_Action."Write", "Script"=w273) -> ()  [unwired: 3 in, 6 out]
                n159 = call "CC System Message.vi"("Message"=w267) -> ()  [unwired: 10 in, 1 out]
              }
              frame "Running", Default {
                n160 = One Button Dialog(message="Cannot take a quick image right now. Image acquisition already underway.") -> ()  [unwired: 1 in, 1 out]
              }
            }
          }
          frame "generate script" {
            # "Name the script file from ID and Obj name"
            # "create the script file and send to script process but don't run it"
            n161 = Unbundle By Name(w293) -> ("Observation List"=w303:T1[], "Row"=w302:i32)
            n162 = property on="Queue" class="MCListbox (strict)"() -> ("ItemSyms"=w307:i32[])  [unwired: 2 in, 2 out]
            n163 = Unbundle By Name(w293) -> ("Script Q"=w285:refnum<queue>)
            n164 = local write "Queue"(w302) -> ()
            n165 = Replace Array Subset(array=w307, new element=4 ("new element/subarray"), index=w302) -> (w305:i32[])
            n166 = Index Array(array=w303, index=w302) -> (element=w286:T1)
            n167 = property on="Queue" class="MCListbox (strict)"("ItemSyms"=w305) -> ()  [unwired: 2 in, 2 out]
            n168 = call "CC Observation to Script.vi"("Observation"=w286) -> ("Script Steps"=w294:T15[])  [unwired: 9 in, 1 out]
            n169 = call "CC Observation Count Images.vi"("element"=w286) -> ("Total Images"=w290:i32)  [unwired: 9 in, 1 out]
            "Queue Running" <- w290
            n170 = Unbundle By Name(w286) -> ("ID"=w300:string)
            n171 = Bundle(cluster=T17 {"Cmd"="", "Parameters"=variant} ("element"), "Cmd"="set observation", "Parameters"=w286) -> (w287:T17)
            n172 = call "Rd Wr Script Defaults.vi"() -> ("Script Settings"=w298:T20)  [unwired: 10 in, 1 out]
            n173 = Format Into String(format string="Obs_%s", w300) -> (resulting string=w284:string)  [unwired: 2 in, 1 out]
            n174 = Enqueue Element(queue=w285, element=w287) -> ()  [unwired: 2 in, 3 out]
            n175 = Unbundle By Name(w298) -> ("Script Path"=w297:path)
            n176 = Bundle By Name(cluster=T14 {"Name"="", "Script"=[]} ("Script"), "Name"=w284, "Script"=w294) -> (w299:T14)
            n177 = Bundle By Name(cluster=w293, "Expected Images"=w290, "script name"=w284) -> (w304:T10)
            n178 = Format Into String(format string="Created script %s.", w284) -> (resulting string=w291:string)  [unwired: 2 in, 1 out]
            n179 = call "CC Rd Wr Script.vi"("Script Path"=w297, "Action"=CC_Rd_Wr_Script_Action."Write", "Script"=w299) -> ()  [unwired: 3 in, 6 out]
            n180 = property on="Queue Running" class="Slide (strict)"("Scale.Maximum"=w290) -> ()  [unwired: 2 in, 2 out]
            n181 = call "CC System Message.vi"("Message"=w291) -> ()  [unwired: 10 in, 1 out]
          }
          frame "start script" {
            # "Wait for script to initialize variables."
            n182 = Unbundle By Name(w316) -> ("Script Q"=w320:refnum<queue>, "script name"=w312:string)
            n183 = Wait (ms)(milliseconds to wait=u32 2000) -> ()  [unwired: 1 out]
            n184 = Bundle By Name(cluster=T17 {"Cmd"="", "Parameters"=variant} ("element"), "Cmd"="set script", "Parameters"=w312) -> (w311:T17)
            n185 = Enqueue Element(queue=w320, element=w311) -> (queue out=w310:refnum<queue>, error out=w308:errorcluster)  [unwired: 2 in, 1 out]
            n186 = Enqueue Element(queue=w310, element=T17 {"Cmd"="start script", "Parameters"=variant}, error in (no error)=w308) -> ()  [unwired: 1 in, 3 out]
            n187 = call "CC System Message.vi"("Message"="Starting Script.") -> ()  [unwired: 10 in, 1 out]
            n188 = Bundle By Name(cluster=w316, "Obs State"=enum16{"Idle", "Running", "Paused"}."Running") -> (w317:T10)
          }
          frame "script complete" {
            n189 = Unbundle By Name(w337) -> ("Row"=w323:i32, "state"=w336:refnum<user-event>, "Observation List"=w324:T1[])
            n190 = Array Size(array=w324) -> (size(s)=w329:i32)
            n191 = Decrement(x=w329) -> (x-1=w328:i32)
            n192 = call "CC System Message.vi"("Message"="Observation Completed.") -> ()  [unwired: 10 in, 1 out]
            n193 = control-ref of="Queue"() -> (w334:refnum<vi>)
            n194 = Less?(x=w323, y=w328) -> (x < y?=w327:bool)
            n195 = property on="Queue" class="MCListbox (strict)"() -> ("ItemSyms"=w342:i32[])  [unwired: 2 in, 2 out]
            n196 = Index Array(array=w324, index=w323) -> (element=w326:T1)
            n197 = Bundle By Name(cluster=w326, "Observation Status"=CC_enum_Observation_Status."Done") -> (w322:T1)
            n198 = And(x=w327, y="Auto Step") -> (x .and. y?=w330:bool)
            n199 = case shown="False" w330 {
              tunnel: w336 -> [w343 w349]
              tunnel: [enum16{"Idle", "Running", "Paused"}."Idle" ("Obs State") enum16{"Idle", "Running", "Paused"}."Running" ("Obs State")] -> w331
              frame False {
                n200 = Generate User Event(user event=w343, event data cluster="queue idle" ("event data")) -> ()  [unwired: 2 in, 2 out]
              }
              frame True {
                n201 = Generate User Event(user event=w349, event data cluster="start queue" ("event data")) -> ()  [unwired: 2 in, 2 out]
                n202 = local write "Queue"(-1 ("Queue")) -> ()
              }
            }
            n203 = Replace Array Subset(array=w342, new element=38 ("new element/subarray"), index=w323) -> (w340:i32[])
            n204 = Replace Array Subset(array=w324, new element=w322, index=w323) -> (w321:T1[])
            n205 = property on="Queue" class="MCListbox (strict)"("ItemSyms"=w340) -> ()  [unwired: 2 in, 2 out]
            n206 = Increment(x=w323) -> (x+1=w339:i32)
            n207 = call "CC Greyout Table Row.vi"("Color"=enum16{"White", "Gray", "Custom"}."Gray", "Row"=w323, "Queue ref"=w334) -> ()  [unwired: 8 in, 1 out]
            n208 = Bundle By Name(cluster=w337, "Row"=w339, "Obs State"=w331, "Observation List"=w321) -> (w338:T10)
          }
          frame "queue idle" {
            w355 = T12."Disabled and Grayed Out" ("Disabled")
            n209 = property on="Queue Running" class="Slide (strict)"("Visible"=FALSE) -> ()  [unwired: 2 in, 2 out]
            n210 = property on="queue idle" class="Str"("Visible"=TRUE) -> ()  [unwired: 2 in, 2 out]
            n211 = One Button Dialog(message="Queued observations completed. Telescope is now idle.") -> ()  [unwired: 1 in, 1 out]
            n212 = property on="Pause Q" class="Bool (strict)"("DisabledEnum"=w355, "Blinking"=FALSE) -> ()  [unwired: 2 in, 2 out]
            n213 = property on="Stop" class="Bool"("DisabledEnum"=w355) -> ()  [unwired: 2 in, 2 out]
            n214 = local write "Queue"(-1 ("Queue")) -> ()
            n215 = property on="Run Queue" class="Bool"("DisabledEnum"=T12."Enabled" ("Disabled")) -> ()  [unwired: 2 in, 2 out]
          }
          frame "script error" {
            n216 = Unbundle By Name(w366) -> ("state"=w365:refnum<user-event>, "Row"=w362:i32, "Observation List"=w363:T1[])
            n217 = property on="Queue" class="MCListbox (strict)"() -> ("ItemSyms"=w372:i32[])  [unwired: 2 in, 2 out]
            n218 = Replace Array Subset(array=w372, new element=2 ("new element/subarray"), index=w362) -> (w370:i32[])
            n219 = Index Array(array=w363, index=w362) -> (element=w360:T1)
            n220 = Bundle By Name(cluster=w360, "Observation Status"=CC_enum_Observation_Status."Error") -> (w359:T1)
            n221 = call "CC System Message.vi"("Message"="Observation Aborted due to error.") -> ()  [unwired: 10 in, 1 out]
            n222 = property on="Queue" class="MCListbox (strict)"("ItemSyms"=w370) -> ()  [unwired: 2 in, 2 out]
            n223 = Generate User Event(user event=w365, event data cluster="queue idle" ("event data")) -> ()  [unwired: 2 in, 2 out]
            n224 = local write "Auto Step"(FALSE ("Auto")) -> ()
            n225 = Replace Array Subset(array=w363, new element=w359, index=w362) -> (w361:T1[])
            n226 = Bundle By Name(cluster=w366, "Obs State"=enum16{"Idle", "Running", "Paused"}."Idle", "Observation List"=w361) -> (w367:T10)
          }
          frame "script abort" {
            n227 = Unbundle By Name(w382) -> ("state"=w381:refnum<user-event>, "Row"=w376:i32, "Observation List"=w375:T1[])
            n228 = local write "Auto Step"(FALSE ("Auto")) -> ()
            n229 = property on="Queue" class="MCListbox (strict)"() -> ("ItemSyms"=w388:i32[])  [unwired: 2 in, 2 out]
            n230 = Index Array(array=w375, index=w376) -> (element=w379:T1)
            n231 = Bundle By Name(cluster=w379, "Observation Status"=CC_enum_Observation_Status."Ready") -> (w378:T1)
            n232 = Replace Array Subset(array=w388, new element=37 ("new element/subarray"), index=w376) -> (w386:i32[])
            n233 = Generate User Event(user event=w381, event data cluster="queue idle" ("event data")) -> ()  [unwired: 2 in, 2 out]
            n234 = property on="Queue" class="MCListbox (strict)"("ItemSyms"=w386) -> ()  [unwired: 2 in, 2 out]
            n235 = Replace Array Subset(array=w375, new element=w378, index=w376) -> (w374:T1[])
            n236 = call "CC System Message.vi"("Message"="Observation Aborted by user") -> ()  [unwired: 10 in, 1 out]
            n237 = Bundle By Name(cluster=w382, "Obs State"=enum16{"Idle", "Running", "Paused"}."Idle", "Observation List"=w374) -> (w383:T10)
          }
          frame "clean table" {
            n238 = control-ref of="Queue"() -> (w391:refnum<vi>)
            n239 = for {
              N: 50 -> [_]
              tunnel: w391 -> [w395]
              i -> [w394]
              n240 = call "CC Greyout Table Row.vi"("Color"=enum16{"White", "Gray", "Custom"}."White", "Row"=w394, "Queue ref"=w395) -> ()  [unwired: 8 in, 1 out]
            }
          }
          frame "shutdown" {
          }
        }
      }
      event "Air Mass Tool": Value Change {
        n241 = event-data() -> ()  [unwired: 1 in, 6 out]
        n242 = Unbundle By Name(w400) -> ("Observation Settings.Air Mass Program Path"=w402:path, "Observation List"=w399:T1[])
        n243 = Empty String/Path?(string/path=w402) -> (empty?=w405:bool)
        n244 = case shown="True" w405 {
          tunnel: [FALSE ("cancelled") w422] -> w404
          tunnel: [w419 w420] -> w403
          tunnel: w402 -> [w419 _]
          frame False {
          }
          frame True {
            n245 = call "File Dialog"() -> ("selected path"=w420:path, "cancelled"=w422:bool, "error out"=w421:errorcluster)  [unwired: 12 in, 1 out]
            n246 = call <vilib>:"Clear Errors.vi"("error in (no error)"=w421) -> ()  [unwired: 5 in, 2 out]
          }
        }
        n247 = case shown="False" w404 {
          tunnel: w403 -> [w413 _]
          tunnel: w400 -> [w410 w417]
          tunnel: [w416 w417] -> w401
          tunnel: w399 -> [w412 _]
          tunnel: "Open Plots" -> [w406 _]
          frame False {
            n248 = call "CC Launch AirMass Calculator.vi"("Show Plots?"=w406, "Observation List"=w412, "AirMass program"=w413) -> ("Air Mass"=w407:T9[], "BlockIDs"=w411:string[])  [unwired: 6 in, 1 out]
            n249 = Unbundle By Name(w410) -> ("state"=w409:refnum<user-event>)
            n250 = Bundle By Name(cluster=w410, "Observation Settings.Air Mass Program Path"=w413, "BlockIDs"=w411, "Air Mass"=w407) -> (w416:T10)
            n251 = Unbundle By Name(w416) -> ("Observation Settings"=w415:T8)
            n252 = Generate User Event(user event=w409, event data cluster="update list" ("event data")) -> ()  [unwired: 2 in, 2 out]
            n253 = call "Rd Wr settings json Observation Settings.vi"("Write? (F:Read)"=TRUE, "Observation Settings"=w415) -> ()  [unwired: 8 in, 2 out]
          }
          frame True {
          }
        }
      }
      event "Queue": Shortcut Menu Activation? {
        n254 = event-data() -> ("MenuRef"=w431:refnum<k9>, "CtlRef"=w435:refnum<vi>, "Coords"=w434:T21)  [unwired: 1 in, 4 out]
        n255 = Unbundle By Name(w432) -> ("Obs State"=w428:enum16{"Idle", "Running", "Paused"}, "Row"=w429:i32, "Observation List"=w427:T1[])
        n256 = invoke class="MCListbox (strict)" method="Point To Row Column"(reference=w435, "Point"=w434) -> ("CellPosition"=w433:T22)  [unwired: 5 in, 6 out]
        n257 = Array Size(array=w427) -> (size(s)=w426:i32)
        n258 = Unbundle By Name(w433) -> ("Row"=w423:i32)
        n259 = Decrement(x=w426) -> (x-1=w424:i32)
        n260 = Equal?(x=w424, y=w423) -> ()  [unwired: 1 out]
        n261 = for {
          tunnel: w431 -> [w442]
          tunnel: string[] ["Move To Top", "Move Up", "Move Down", "Move to Bottom", "Remove from Queue", "Clear Completed", "Clear All"] -> [w441] mode=indexing
          tunnel: w429 -> [w439]
          tunnel: w423 -> [w438]
          tunnel: w428 -> [w437]
          tunnel: w424 -> [w436]
          n262 = case shown="\"Running\", Default" w437 {
            tunnel: w441 -> [w447 w477]
            tunnel: [w446 w476] -> w440
            tunnel: w439 -> [w445 w475]
            tunnel: w438 -> [w444 w474]
            tunnel: w436 -> [w443 w473]
            frame "Running", Default {
              n263 = case shown="\"Move To Top\"" w447 {
                tunnel: [TRUE w449 w453 w457 w463 w468 TRUE FALSE] -> w446
                tunnel: w445 -> [_ w451 w455 w460 w466 w469 _ _]
                tunnel: w444 -> [_ w450 w454 w459 w465 w470 _ _]
                tunnel: w443 -> [_ _ _ w458 w464 _ _ _]
                frame "False", Default {
                }
                frame "Move To Top" {
                  n264 = Less?(x=w451, y=w450) -> (x < y?=w449:bool)
                }
                frame "Move Up" {
                  n265 = Increment(x=w455) -> (x+1=w452:i32)
                  n266 = Less?(x=w452, y=w454) -> (x < y?=w453:bool)
                }
                frame "Move Down" {
                  n267 = Less?(x=w460, y=w459) -> (x < y?=w461:bool)
                  n268 = Less?(x=w459, y=w458) -> (x < y?=w456:bool)
                  n269 = And(x=w461, y=w456) -> (x .and. y?=w457:bool)
                }
                frame "Move to Bottom" {
                  n270 = Less?(x=w466, y=w465) -> (x < y?=w467:bool)
                  n271 = Less?(x=w465, y=w464) -> (x < y?=w462:bool)
                  n272 = And(x=w467, y=w462) -> (x .and. y?=w463:bool)
                }
                frame "Remove from Queue" {
                  n273 = Not Equal?(x=w469, y=w470) -> (x != y?=w468:bool)
                }
                frame "Clear Completed" {
                }
                frame "Clear All" {
                }
              }
            }
            frame "Idle" {
              n274 = case shown="\"Move To Top\"" w477 {
                tunnel: [TRUE TRUE w481 w483 w489 TRUE TRUE TRUE] -> w476
                tunnel: w475 -> [_ _ w480 w486 w492 _ _ _]
                tunnel: w474 -> [_ _ w482 w485 w491 _ _ _]
                tunnel: w473 -> [_ _ _ w484 w490 _ _ _]
                frame "False", Default {
                }
                frame "Move To Top" {
                }
                frame "Move Up" {
                  n275 = Less?(x=w480, y=w482) -> (x < y?=w481:bool)
                }
                frame "Move Down" {
                  n276 = Less?(x=w486, y=w485) -> (x < y?=w488:bool)
                  n277 = Less?(x=w485, y=w484) -> (x < y?=w487:bool)
                  n278 = And(x=w488, y=w487) -> (x .and. y?=w483:bool)
                }
                frame "Move to Bottom" {
                  n279 = Less?(x=w492, y=w491) -> (x < y?=w494:bool)
                  n280 = Less?(x=w491, y=w490) -> (x < y?=w493:bool)
                  n281 = And(x=w494, y=w493) -> (x .and. y?=w489:bool)
                }
                frame "Remove from Queue" {
                }
                frame "Clear Completed" {
                }
                frame "Clear All" {
                }
              }
            }
          }
          n282 = Set Menu Item Info(7:w441, 9:w440, 11:w442) -> ()  [unwired: 4 in, 2 out]
        }
        n283 = event-data("Discard?"=FALSE) -> ()  [unwired: 1 in, 1 out]
      }
      event "Queue": Shortcut Menu Selection (User) {
        n284 = event-data() -> ("CtlRef"=w513:refnum<vi>, "ItemTag"=w514:string, "Coords"=w512:T21)  [unwired: 1 in, 2 out]
        n285 = Unbundle By Name(w501) -> ("state"=w498:refnum<user-event>, "Observation List"=w510:T1[], "Row"=w506:i32, "Obs State"=w509:enum16{"Idle", "Running", "Paused"})
        n286 = invoke class="MCListbox (strict)" method="Point To Row Column"(reference=w513, "Point"=w512) -> ("CellPosition"=w511:T22)  [unwired: 5 in, 6 out]
        n287 = Equal?(x=w509, y=enum16{"Idle", "Running", "Paused"}."Idle") -> (x = y?=w507:bool)
        n288 = Increment(x=w506) -> (x+1=w505:i32)
        n289 = Generate User Event(user event=w498, event data cluster="update list" ("event data")) -> ()  [unwired: 2 in, 2 out]
        n290 = Select(t=w506, s=w507, f=w505) -> (s? t:f=w504:i32)
        n291 = case shown="\"Remove from Queue\"" w514 {
          tunnel: w511 -> [_ w524 w530 w545 w551 w562 _ _]
          tunnel: w510 -> [w516 w523 w532 w536 w552 w561 w567 _]
          tunnel: w506 -> [w515 w517 w525 w534 w546 w557 w564 _]
          tunnel: w504 -> [_ w519 _ _ _ _ _ _]
          tunnel: [w516 w518 w526 w535 w547 w555 w566 _] -> w503
          tunnel: [w515 w517 w525 w534 w546 w553 w563 0 ("Row")] -> w500
          frame "False", Default {
          }
          frame "Move To Top" {
            n292 = Unbundle By Name(w524) -> ("Row"=w522:i32)
            n293 = Delete From Array(array=w523, index=w522) -> (deleted portion=w520:T1, array with subset deleted=w521:T1[])  [unwired: 1 in]
            n294 = Insert Into Array(array=w521, index=w519, new element=w520) -> (w518:T1[])
          }
          frame "Move Up" {
            n295 = Unbundle By Name(w530) -> ("Row"=w528:i32)
            n296 = Delete From Array(array=w532, index=w528) -> (deleted portion=w529:T1, array with subset deleted=w531:T1[])  [unwired: 1 in]
            n297 = Decrement(x=w528) -> (x-1=w527:i32)
            n298 = Insert Into Array(array=w531, index=w527, new element=w529) -> (w526:T1[])
          }
          frame "Move Down" {
            n299 = Unbundle By Name(w545) -> ("Row"=w539:i32)
            n300 = Array Size(array=w536) -> (size(s)=w541:i32)
            n301 = Index Array(array=w536, index=w539) -> (element=w544:T1)
            n302 = Decrement(x=w541) -> (x-1=w540:i32)
            n303 = Add(x=2, y=w539) -> (x+y=w543:i32)
            n304 = Less Or Equal?(x=w540, y=w539) -> (x <= y?=w538:bool)
            n305 = Insert Into Array(array=w536, index=w543, new element=w544) -> (w542:T1[])
            n306 = Delete From Array(array=w542, index=w539) -> (array with subset deleted=w537:T1[])  [unwired: 1 in, 1 out]
            n307 = Select(t=w536, s=w538, f=w537) -> (s? t:f=w535:T1[])
          }
          frame "Move to Bottom" {
            n308 = Unbundle By Name(w551) -> ("Row"=w550:i32)
            n309 = Delete From Array(array=w552, index=w550) -> (deleted portion=w548:T1, array with subset deleted=w549:T1[])  [unwired: 1 in]
            n310 = Build Array (concatenate)(w549, w548) -> (w547:T1[])
          }
          frame "Remove from Queue" {
            n311 = Unbundle By Name(w562) -> ("Row"=w560:i32)
            n312 = Greater Or Equal?(x=w557, y=w560) -> (x >= y?=w559:bool)
            n313 = Delete From Array(array=w561, index=w560) -> (array with subset deleted=w555:T1[])  [unwired: 1 in, 1 out]
            n314 = Decrement(x=w557) -> (x-1=w558:i32)
            n315 = Select(t=w558, s=w559, f=w557) -> (s? t:f=w556:i32)
            n316 = Max & Min(x=0, y=w556) -> (max(x,y)=w553:i32)  [unwired: 1 out]
            n317 = local write "Queue"(w553) -> ()
          }
          frame "Clear Completed" {
            w563 = 0 ("Row")
            n318 = control-ref of="Queue"() -> (w565:refnum<vi>)
            n319 = Split 1D Array(array=w567, index=w564) -> (second subarray=w566:T1[])  [unwired: 1 out]
            n320 = for {
              N: w564 -> [_]
              tunnel: w565 -> [w570]
              i -> [w569]
              n321 = call "CC Greyout Table Row.vi"("Color"=enum16{"White", "Gray", "Custom"}."White", "Row"=w569, "Queue ref"=w570) -> ()  [unwired: 8 in, 1 out]
            }
            n322 = local write "Queue"(w563) -> ()
          }
          frame "Clear All" {
          }
        }
        n323 = Bundle By Name(cluster=w501, "Observation List"=w503, "Row"=w500) -> (w502:T10)
      }
      event "Run Queue": Value Change {
        n324 = event-data() -> ()  [unwired: 1 in, 1 out]
        n325 = Unbundle By Name(w578) -> ("state"=w577:refnum<user-event>)
        n326 = call "CC Alarm Object.vi"("Alarm Action"=CC_enum_Alarm_Action."Get Alarms") -> ("Alarm List"=w574:T23[], "Alarm?"=w575:bool)  [unwired: 7 in, 2 out]
        n327 = Index Array(array=w574) -> (element=w573:T23)  [unwired: 1 in]
        n328 = Unbundle By Name(w573) -> ("Message"=w572:string)
        n329 = case shown="True" w575 {
          tunnel: w577 -> [w580 _]
          tunnel: w572 -> [_ w581]
          frame False {
            n330 = Generate User Event(user event=w580, event data cluster="start queue" ("event data")) -> ()  [unwired: 2 in, 2 out]
          }
          frame True {
            n331 = Format Into String(format string="Alarm condition prevents observations. Clear alarm and try again.\n\nAlarm message: %s" ("message"), w581) -> (resulting string=w583:string)  [unwired: 2 in, 1 out]
            n332 = One Button Dialog(message=w583) -> ()  [unwired: 1 in, 1 out]
          }
        }
      }
      event "Pause Q": Value Change {
        # "send pause or resume"
        # "Send command to pause after complete of the current step in the script"
        n333 = event-data() -> ()  [unwired: 1 in, 6 out]
        n334 = Unbundle By Name(w589) -> ("Script Q"=w588:refnum<queue>)
        n335 = Select(t=T17 {"Cmd"="pause", "Parameters"=variant} ("element"), s="Pause Q", f=T17 {"Cmd"="resume", "Parameters"=variant} ("element")) -> (s? t:f=w584:T17)
        n336 = Enqueue Element(queue=w588, element=w584) -> ()  [unwired: 2 in, 3 out]
      }
      event "Stop": Value Change {
        # "Send abort script command."
        n337 = event-data() -> ()  [unwired: 1 in, 6 out]
        n338 = Unbundle By Name(w594) -> ("state"=w591:refnum<user-event>, "Script Q"=w593:refnum<queue>)
        n339 = Enqueue Element(queue=w593, element=T17 {"Cmd"="abort script", "Parameters"=variant}) -> ()  [unwired: 2 in, 3 out]
        n340 = local write "Auto Step"(FALSE ("Auto")) -> ()
        n341 = Generate User Event(user event=w591, event data cluster="script abort" ("event data")) -> ()  [unwired: 2 in, 2 out]
      }
      event "clean table": Value Change {
        n342 = event-data() -> ()  [unwired: 1 in, 6 out]
        n343 = Unbundle By Name(w598) -> ("state"=w597:refnum<user-event>)
        n344 = Generate User Event(user event=w597, event data cluster="clean table" ("event data")) -> ()  [unwired: 2 in, 2 out]
      }
      event "Close": Value Change {
        n345 = event-data() -> ()  [unwired: 1 in, 2 out]
      }
    }
  }
